vi "Turbo go for State.vi"(4 "Publish? (T)":bool=TRUE, 6 "Really? (T)":bool=TRUE, 7 "Immediately (false = stick to schedule)":bool, 8 "error in (no error)":errorcluster, 9 "State Timeout (Inf=no timeout )":dbl=inf, 10 "Turbo State":T1=enum."Idle", 11 "Turbo in":refnum<class "Turbo.lvclass">) -> (0 "error out":errorcluster, 3 "Turbo out":refnum<class "Turbo.lvclass">)   [LabVIEW 2015, in "cRIO-Carbondioxide.lvlib" / "CO2-Actor.lvlib" / "Turbo.lvclass"]
uses:
  Turbo.lvclass
  Turbo State Enumerator.ctl
  Turbo.lvclass/Turbo.ctl
  <vilib>/ActorFramework/Time-Delayed Send Message/Time-Delay Override Options.ctl
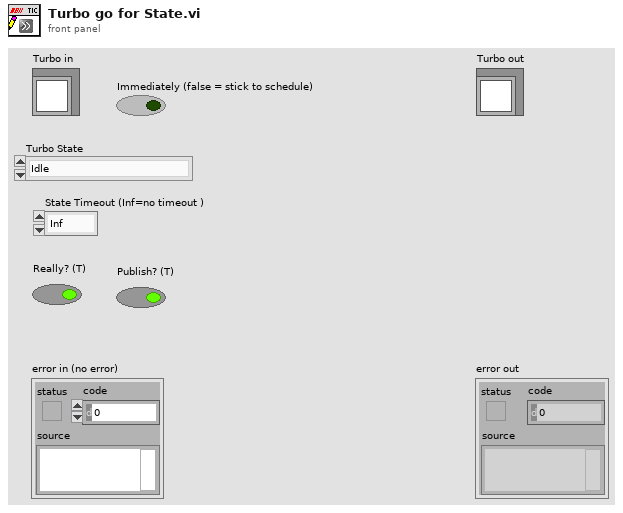
[diagram p1: front panel]
types:
  T1 = typedef "cRIO-Carbondioxide.lvlib/CO2-Actor.lvlib/Turbo.lvclass/Turbo State Enumerator.ctl" = enum16{"Undefined", "Error", "Abort", "Idle", "Initialize", "Start FV Pump", "Wait on FV Gauge", "Start Turbo", "Running", "Stop"}
  T2 = typedef "Time-Delay Override Options.ctl" = enum16{"Send next copy now", "Skip next scheduled copy", "Send next copy now and stop all further copies", "Stop all further copies"}
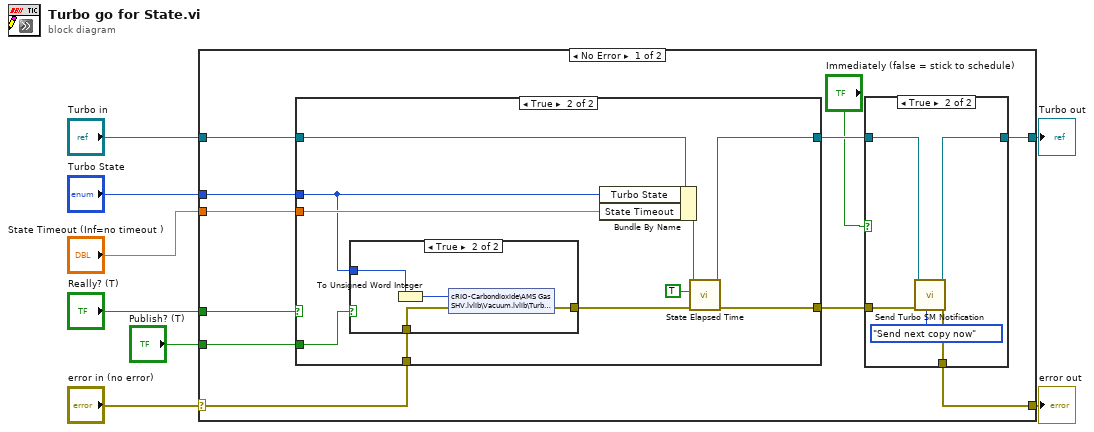
[diagram p0: block diagram]
diagram:
  n1 = case shown="No Error" "error in (no error)" {
    selector: "error in (no error)" -> [w19 w44]
    tunnel: [w12 w44] -> w7
    tunnel: [w11 w45] -> w5
    tunnel: "Turbo in" -> [w17 w45]
    tunnel: "Turbo State" -> [w18 _]
    tunnel: "State Timeout (Inf=no timeout )" -> [w16 _]
    tunnel: "Really? (T)" -> [w15 _]
    tunnel: "Publish? (T)" -> [w14 _]
    frame No Error {
      n2 = case shown="True" w15 {
        tunnel: w19 -> [w28 w38]
        tunnel: w18 -> [_ w33]
        tunnel: w17 -> [w27 w30]
        tunnel: w16 -> [_ w37]
        tunnel: w14 -> [_ w32]
        tunnel: [w28 w31] -> w13
        tunnel: [w27 w29] -> w10
        frame False {
        }
        frame True {
          n3 = case shown="True" w32 {
            tunnel: w38 -> [w39 w42]
            tunnel: [w39 w40] -> w36
            tunnel: w33 -> [_ w43]
            frame False {
            }
            frame True {
              n4 = To Unsigned Word Integer(number=w43) -> (unsigned 16bit integer=w41:u16)
              n5 = shared-variable "cRIO-Carbondioxide\\AMS Gas SHV.lvlib\\Vacuum.lvlib\\Turbo State"(w41, error in=w42) -> (error out=w40:errorcluster)
            }
          }
          n6 = Bundle By Name(cluster=w30, "Turbo State"=w33, "State Timeout"=w37) -> (w35:refnum<class "Turbo.lvclass">)
          n7 = call "State Elapsed Time.vi"("error in (no error)"=w36, "Reset (F)"=TRUE, "Turbo in"=w35) -> ("error out"=w31:errorcluster, "Turbo out"=w29:refnum<class "Turbo.lvclass">)  [unwired: 5 in, 2 out]
        }
      }
      n8 = case shown="True" "Immediately (false = stick to schedule)" {
        tunnel: w13 -> [w20 w26]
        tunnel: [w20 w25] -> w12
        tunnel: [w21 w24] -> w11
        tunnel: w10 -> [w21 w23]
        frame False {
        }
        frame True {
          n9 = call "Send Turbo SM Notification.vi"("notification (Send next copy now)"=Time-Delay_Override_Options."Send next copy now", "error in (no error)"=w26, "Turbo in"=w23) -> ("error out"=w25:errorcluster, "Turbo out"=w24:refnum<class "Turbo.lvclass">)  [unwired: 7 in]
        }
      }
    }
    frame Error {
    }
  }
  "error out" <- w7
  "Turbo out" <- w5
